vi "Read Service Information.vi"(8 "error in (no error)":errorcluster, 11 "Lotis in":refnum<class "PL Lotis TII LS.lvclass">) -> (0 "error out":errorcluster, 2 "information":T1, 3 "Lotis out":refnum<class "PL Lotis TII LS.lvclass">)   [LabVIEW 2015, in "PL Lotis TII LS.lvclass"]
doc: "Reads service information."
uses:
  PL Lotis TII LS.lvclass
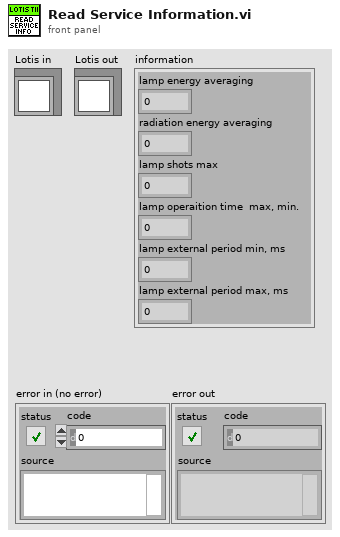
[diagram p1: front panel]
types:
  T1 = cluster{"lamp energy averaging":u32, "radiation energy averaging":u32, "lamp shots max":u32, "lamp operaition time  max, min.":u32, "lamp external period min, ms":u32, "lamp external period max, ms":u32}
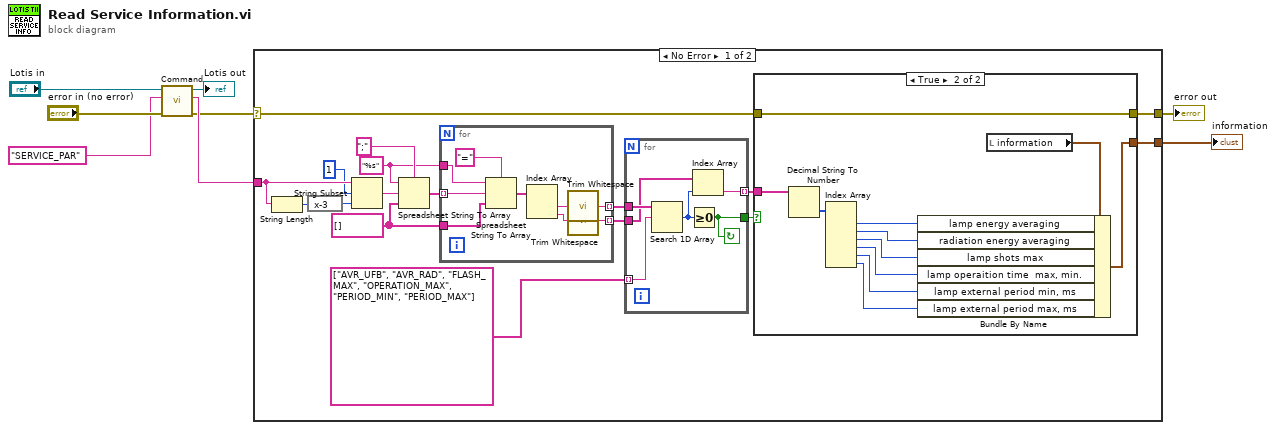
[diagram p0: block diagram]
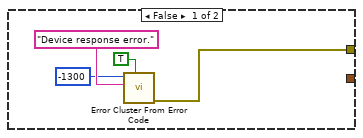
[diagram p2: hidden frame]
diagram:
  n1 = call "Command.vi"("error in (no error)"="error in (no error)", "command"="SERVICE_PAR", "Lotis in"="Lotis in") -> ("error out"=w3:errorcluster, "response data"=w4:string, "Lotis out"=→"Lotis out":refnum<class "PL Lotis TII LS.lvclass">)  [unwired: 6 in]
  n2 = case shown="No Error" w3 {
    selector: w3 -> [w14 w56]
    tunnel: w4 -> [w25 _]
    tunnel: [w13 w56] -> w2
    tunnel: [w9 _] -> w1
    frame No Error {
      w18 = "%s" ("format string")
      w17 = string[] [] ("array type (2D Dbl)")
      n3 = String Length(string=w25) -> (length=w23:i32)
      n4 = expression code="x-3"(w23) -> (w22:i32)
      n5 = String Subset(string=w25, offset (0)=1, length (rest)=w22) -> (substring=w21:string)
      n6 = Spreadsheet String To Array(delimiter (Tab)=";", format string=w18, spreadsheet string=w21, array type (2D Dbl)=w17) -> (array=w19:string[])
      n7 = for {
        tunnel: w19 -> [w52] mode=indexing
        tunnel: w18 -> [w55]
        tunnel: w17 -> [w53]
        tunnel: [w48] -> w16 mode=indexing
        tunnel: [w47] -> w11 mode=indexing
        n8 = Spreadsheet String To Array(delimiter (Tab)="=", format string=w55, spreadsheet string=w52, array type (2D Dbl)=w53) -> (array=w51:string[])
        n9 = Index Array(array=w51) -> (element #1=w50:string, element #2=w49:string)  [unwired: 2 in]
        n10 = call <vilib>:"Trim Whitespace.vi"("string"=w50) -> ("trimmed string"=w48:string)  [unwired: 1 in]
        n11 = call <vilib>:"Trim Whitespace.vi"("string"=w49) -> ("trimmed string"=w47:string)  [unwired: 1 in]
      }
      n12 = for {
        tunnel: w16 -> [w46]
        tunnel: string[] ["AVR_UFB", "AVR_RAD", "FLASH_MAX", "OPERATION_MAX", "PERIOD_MIN", "PERIOD_MAX"] -> [w45] mode=indexing
        tunnel: [w44] -> w12
        tunnel: w11 -> [w43]
        tunnel: [w41] -> w10 mode=indexing
        stop <- w44 continue-if-true
        n13 = Search 1D Array(1D array=w46, element=w45) -> (index of element=w42:i32)  [unwired: 1 in]
        n14 = Greater Or Equal To 0?(x=w42) -> (x >= 0?=w44:bool)
        n15 = Index Array(array=w43, index=w42) -> (element=w41:string)
      }
      n16 = case shown="True" w12 {
        tunnel: w14 -> [_ w40]
        tunnel: [w26 w40] -> w13
        tunnel: w10 -> [_ w37]
        tunnel: [_ w38] -> w9
        frame False {
          n17 = call <vilib>:"Error Cluster From Error Code.vi"("show call chain? (False)"=TRUE, "error message (\"\")"="Device response error." ("format string"), "error code (0)"=-1300) -> ("error out"=w26:errorcluster)  [unwired: 6 in]
        }
        frame True {
          n18 = Decimal String To Number(string=w37) -> (number=w36:i32[])  [unwired: 2 in, 1 out]
          n19 = Index Array(array=w36) -> (element #1=w35:i32, element #2=w34:i32, element #3=w33:i32, element #4=w32:i32, element #5=w31:i32, element #6=w30:i32)  [unwired: 6 in]
          n20 = local read "information"() -> (w39:T1)
          n21 = Bundle By Name(cluster=w39, "lamp energy averaging"=w35, "radiation energy averaging"=w34, "lamp shots max"=w33, "lamp operaition time  max, min."=w32, "lamp external period min, ms"=w31, "lamp external period max, ms"=w30) -> (w38:T1)
        }
      }
    }
    frame Error {
    }
  }
  "error out" <- w2
  "information" <- w1
